vi "Set Folders.vi"(8 "error in (no error)":errorcluster, 9 "Data folder":path, 10 "Calibration folder":path, 11 "Tosca in":refnum<class "Parameters.lvclass">) -> (0 "error out":errorcluster, 3 "Tosca out":refnum<class "Parameters.lvclass">)   [LabVIEW 2015, in "Parameters.lvclass"]
uses:
  Parameters.lvclass
  Parameters.lvclass/Parameters.ctl
  State/State.lvclass
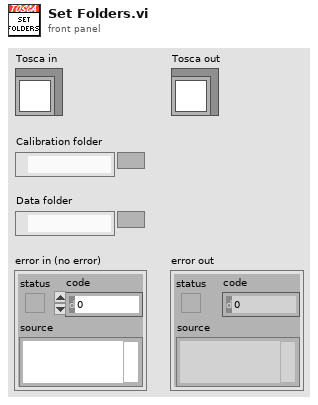
[diagram p1: front panel]
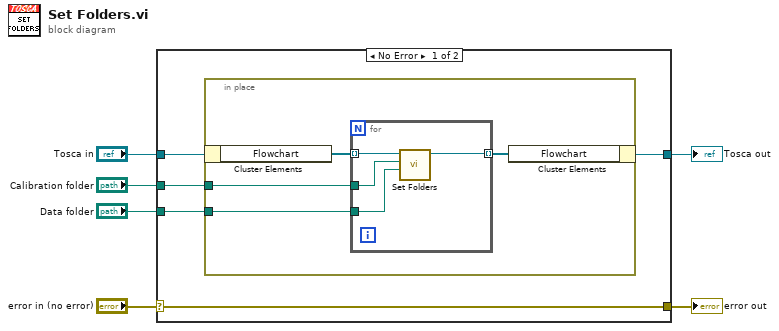
[diagram p0: block diagram]
diagram:
  n1 = case shown="No Error" "error in (no error)" {
    selector: "error in (no error)" -> [w11 w21]
    tunnel: [w11 w21] -> w5
    tunnel: [w9 w20] -> w3
    tunnel: "Tosca in" -> [w10 w20]
    tunnel: "Calibration folder" -> [w8 _]
    tunnel: "Data folder" -> [w7 _]
    frame No Error {
      n2 = in-place {
        in-place-border: w8 -> [w13]
        in-place-border: w7 -> [w12]
        n3 = in-place-cluster #1(w10) -> ("Flowchart"=w15:refnum<class "State.lvclass">[])
        n4 = for {
          tunnel: w15 -> [w19] mode=indexing
          tunnel: [w18] -> w14 mode=indexing
          tunnel: w13 -> [w17]
          tunnel: w12 -> [w16]
          n5 = call "Set Folders.vi"("Data folder"=w16, "Calibration folder"=w17, "State in"=w19) -> ("State out"=w18:refnum<class "State.lvclass">)  [unwired: 7 in, 1 out]
        }
        n6 = in-place-cluster #1("Flowchart"=w14) -> (w9:refnum<class "Parameters.lvclass">)
      }
    }
    frame Error {
    }
  }
  "error out" <- w5
  "Tosca out" <- w3
